vi "Wait.vi"(11 "Time":dbl) -> ()   [LabVIEW 2020]
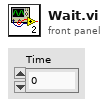
[diagram p1: front panel]
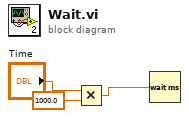
[diagram p0: block diagram]
diagram:
  n1 = Multiply(x="Time", y=1000.0) -> (x*y=w1:dbl)
  n2 = Wait (ms)(milliseconds to wait=w1) -> ()  [unwired: 1 out]
